vi "Problem1.8.vi"() -> ()   [LabVIEW 2019]
panel:
  out "Random Number Array":dbl[](array[numeric])
  out "Histogram":dynamicdata(graph)
  out "Uniform Deviate Array":dbl[](array[numeric])
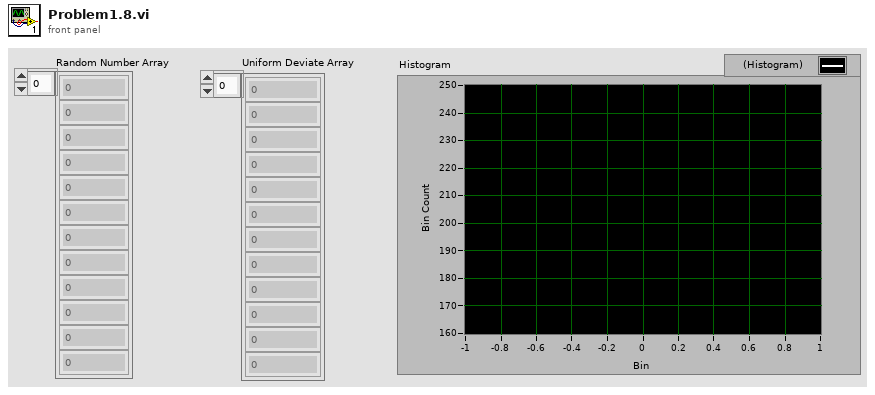
[diagram p1: front panel]
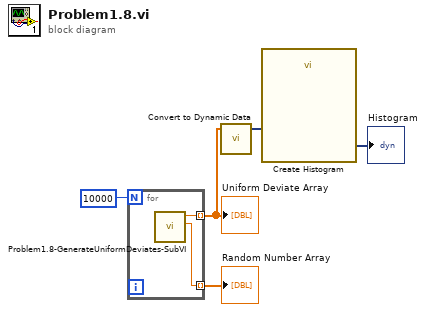
[diagram p0: block diagram]
diagram:
  n1 = for {
    N: 10000 -> [_]
    tunnel: [w7] -> w2 mode=indexing
    tunnel: [w6] -> w1 mode=indexing
    n2 = call "Problem1.8-GenerateUniformDeviates-SubVI.vi"() -> ("number: 0 to 1"=w6:dbl, "Numeric"=w7:dbl)  [unwired: 10 in]
  }
  "Uniform Deviate Array" <- w2
  "Random Number Array" <- w1
  n3 = call "Convert to Dynamic Data"("Array"=w2) -> ("Dynamic Data Type"=w4:dynamicdata)  [unwired: 3 in]
  n4 = call "Create Histogram"("Signal"=w4) -> ("Histogram"=→"Histogram":dynamicdata)  [unwired: 9 in, 1 out]
